vi "Problem 24.vi"() -> ()   [LabVIEW 2013, in "Problem 24.lvlib"]
uses:
  Problem 24.lvlib
panel:
  out "Millionth Lexicograph Permutation":string
  out "Lexicographic Permutations":string[](array[string])
  in  "Array to Permutate":string[](array[string])=["0", "1", "2", "3", "4", "5", "6", "7", "8", "9"]
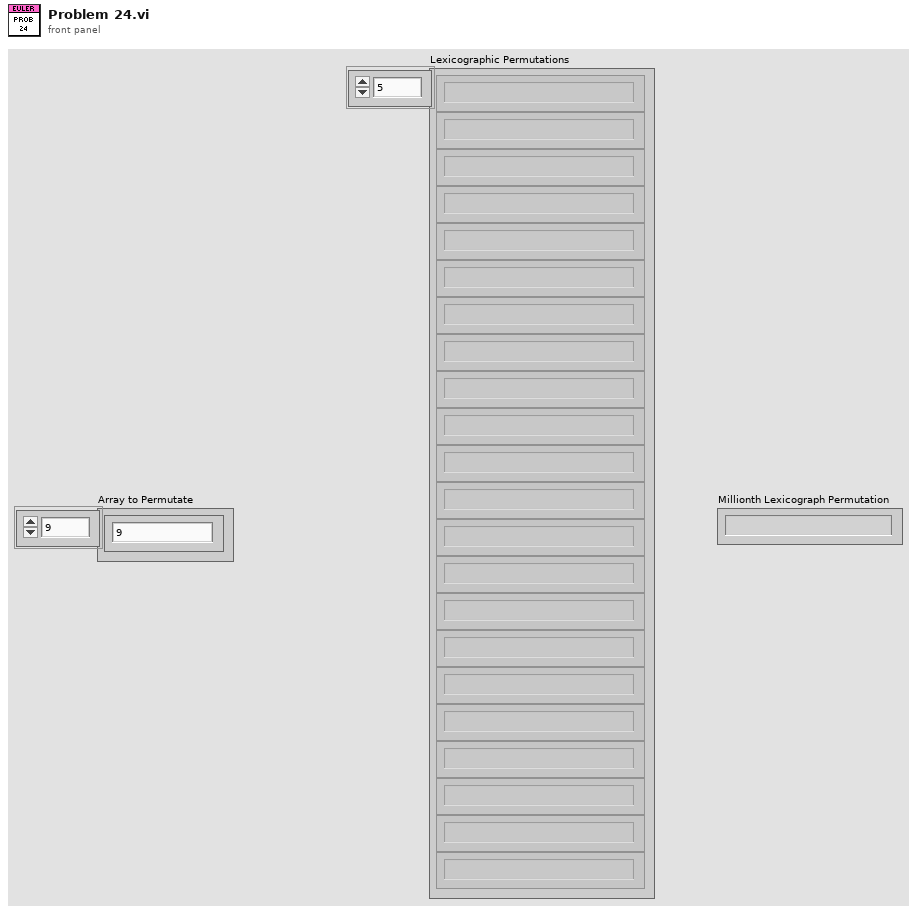
[diagram p1: front panel]
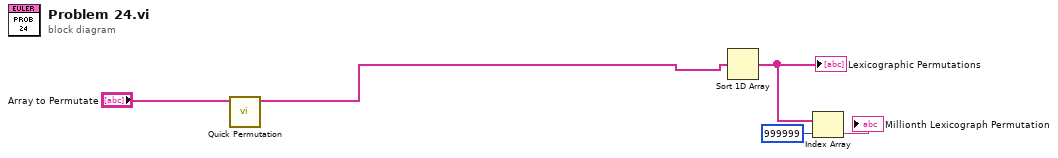
[diagram p0: block diagram]
diagram:
  n1 = call "Quick Permutation.vi"("Array to Permutate"="Array to Permutate") -> ("Permutations"=w1:string[])  [unwired: 9 in, 1 out]
  n2 = Sort 1D Array(array=w1) -> (sorted array=w4:string[])
  "Lexicographic Permutations" <- w4
  n3 = Index Array(array=w4, index=999999) -> (element=→"Millionth Lexicograph Permutation":string)
